vi "Get Port.vi"(8 "error in (no error)":errorcluster, 11 "Network Config in":refnum<class "Network Config.lvclass">) -> (0 "error out":errorcluster, 2 "Port":u16, 3 "Network Config out":refnum<class "Network Config.lvclass">)   [LabVIEW 2020, in "Examples.lvlib" / "Network Config.lvclass"]
uses:
  Network Config.lvclass
  Network Config.lvclass/Network Config.ctl
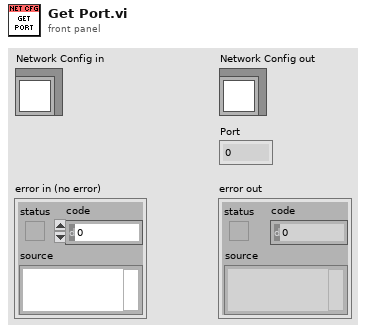
[diagram p1: front panel]
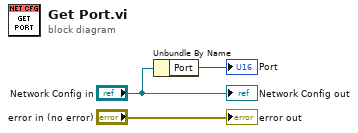
[diagram p0: block diagram]
diagram:
  n1 = Unbundle By Name("Network Config in") -> ("Port"=→"Port":u16)
  "error out" <- "error in (no error)"
  "Network Config out" <- "Network Config in"
